vi "Parse URI.vi"(0 "URI":string="ws://hostname.domain:80/resource/name", 7 "URI type (WS)":enum16{"WS", "HTTP"}(ring), 11 "error in":errorcluster) -> (3 "Secure":bool, 4 "URI Out":string="ws://hostname.domain:80/resource/name", 6 "Hostname":string, 8 "HTTP URI":string, 10 "Resource Name":string, 13 "Port":u16, 14 "Default Port":bool, 15 "error out":errorcluster)   [LabVIEW 2021, in "LV WebSockets.lvlib"]
doc: "Parses a websocket or HTTP URI and outputs its components"
uses:
  LV WebSockets.lvlib
  <vilib>/Utility/error.llb/Error Cluster From Error Code.vi
  <vilib>/regexp/Match Regular Expression.xnode
  <vilib>/ErrorRing/Error Ring.xnode
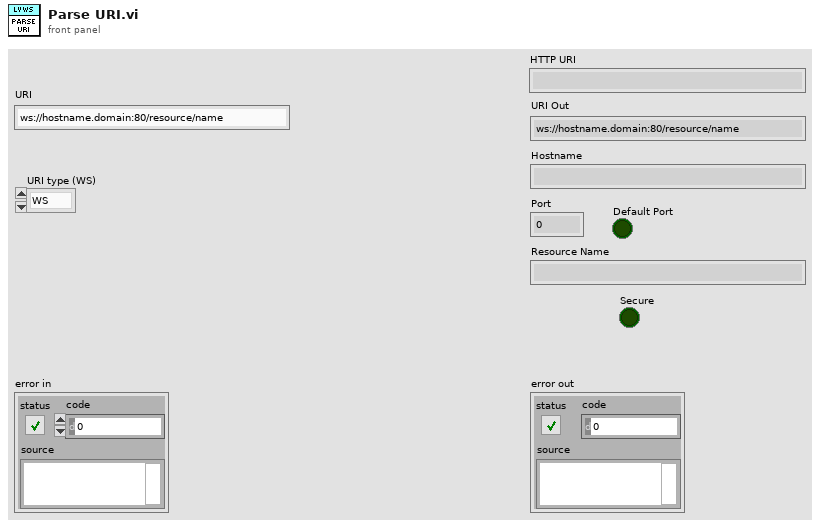
[diagram p1: front panel]
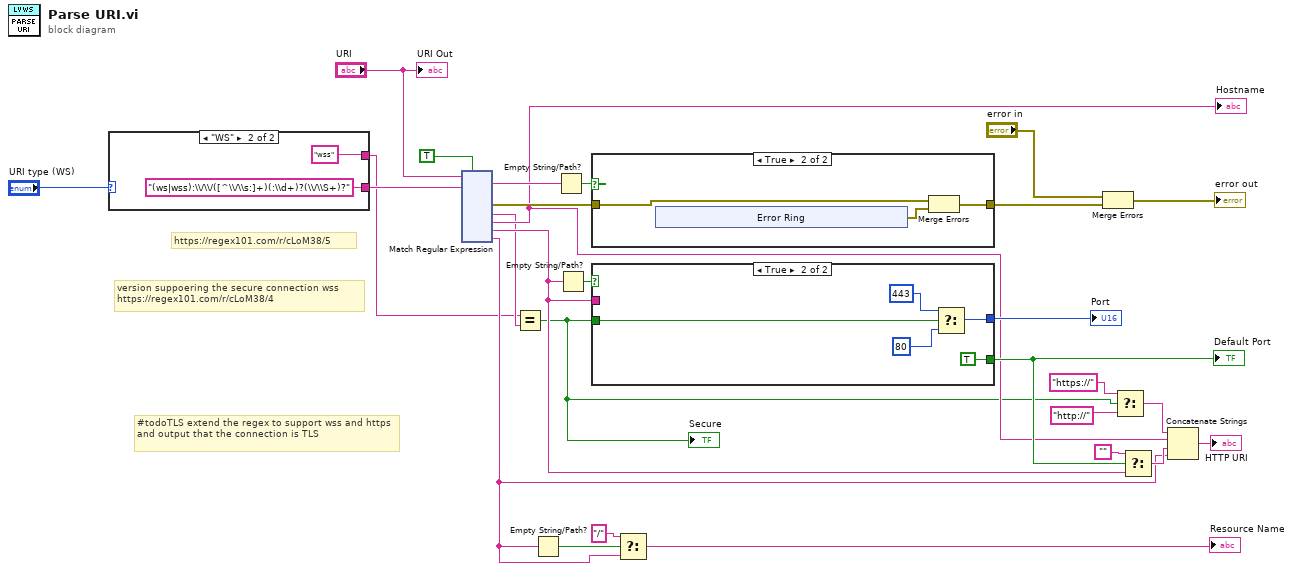
[diagram p0: block diagram]
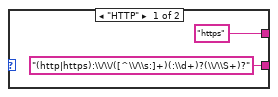
[diagram p2: hidden frame]
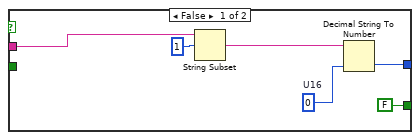
[diagram p4: hidden frame]
diagram:
  # "version suppoering the secure connection wss \nhttps://regex101.com/r/cLoM38/4"
  # "#todoTLS extend the regex to support wss and https and output that the connection is TLS"
  # "https://regex101.com/r/cLoM38/5"
  n1 = case shown="\"WS\"" "URI type (WS)" {
    tunnel: ["(http|https):\\/\\/([^\\/\\s:]+)(:\\d+)?(\\/\\S+)?" ("regular expression") "(ws|wss):\\/\\/([^\\/\\s:]+)(:\\d+)?(\\/\\S+)?" ("regular expression")] -> w27
    tunnel: ["https" ("regular expression") "wss" ("regular expression")] -> w5
    frame "HTTP" {
    }
    frame "WS" {
    }
  }
  n2 = xnode "Match Regular Expression"("input string"="URI", "regular expression"=w27, "ignore case? (F)"=TRUE) -> ("whole match"=w23:string, "error out"=w20:errorcluster, "submatch 1"=w6:string, "submatch 2"=w7:string, "submatch 3"=w8:string, "submatch 4"=w9:string)  [unwired: 3 in, 3 out]
  "Hostname" <- w7
  n3 = Equal?(x=w5, y=w6) -> (x = y?=w1:bool)
  "Secure" <- w1
  n4 = Empty String/Path?(string/path=w9) -> (empty?=w17:bool)
  n5 = Empty String/Path?(string/path=w23) -> (empty?=w21:bool)
  n6 = Empty String/Path?(string/path=w8) -> (empty?=w26:bool)
  n7 = case shown="True" w21 {
    tunnel: w20 -> [w33 w36]
    tunnel: [w33 w34] -> w19
    frame False {
    }
    frame True {
      n8 = xnode ("Error Ring")() -> ("error out"=w35:errorcluster)
      n9 = Merge Errors(w36, w35) -> (w34:errorcluster)
    }
  }
  n10 = case shown="True" w26 {
    tunnel: w8 -> [w44 _]
    tunnel: [w43 w51] -> w25
    tunnel: [FALSE TRUE] -> w14
    tunnel: w1 -> [_ w48]
    frame False {
      w45 = u16 0  # U16
      n11 = String Subset(string=w44, offset (0)=1) -> (substring=w46:string)  [unwired: 1 in]
      n12 = Decimal String To Number(string=w46, default (0L)=w45) -> (number=w43:u16)  [unwired: 1 in, 1 out]
    }
    frame True {
      n13 = Select(t=u16 443, s=w48, f=u16 80) -> (s? t:f=w51:u16)
    }
  }
  "Default Port" <- w14
  "Port" <- w25
  n14 = Select(t="/", s=w17, f=w9) -> (s? t:f=→"Resource Name":string)
  n15 = Merge Errors("error in", w19) -> (→"error out":errorcluster)
  n16 = Select(t="https://" ("string"), s=w1, f="http://" ("string")) -> (s? t:f=w2:string)
  n17 = Select(t="", s=w14, f=w8) -> (s? t:f=w12:string)
  n18 = Concatenate Strings(w2, w7, w12, w9) -> (→"HTTP URI":string)
  "URI Out" <- "URI"
